vi "Degrees to Arc Length.vi"(5 "Angle":dbl) -> (2 "Arc Length (inches)":dbl)   [LabVIEW 2014]
uses:
  global variables/robot_const.vi
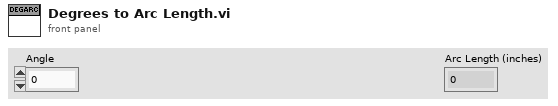
[diagram p1: front panel]
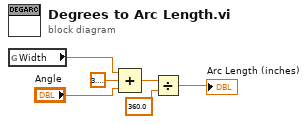
[diagram p0: block diagram]
diagram:
  n1 = global read "robot_const.vi" "Width"() -> (w4:dbl)
  n2 = Compound Arithmetic op=ADD(w4, 3.141592653589793, "Angle") -> (w3:dbl)
  n3 = Divide(x=w3, y=360.0) -> (x/y=→"Arc Length (inches)":dbl)
